vi "Mail整体图.vi"() -> ()   [LabVIEW 2014]
panel:
  in  "Check":bool
  in  "Unsubscribe":bool
  in  "Subscribe":bool
  in  "Signature":bool
  in  "Sign":bool
  in  "Send":bool
  in  "Reply":bool
  in  "Reply all":bool
  in  "Queue":bool
  in  "Post":bool
  in  "Node":bool
  in  "News":bool
  in  "New":bool
  in  "New font":bool
  in  "Mailbox":bool
  in  "Mail":bool
  in  "Log":bool
  in  "Get":bool
  in  "Generic":bool
  in  "Forward":bool
  in  "Fonts":bool
  in  "Find":bool
  in  "Email":bool
  in  "Delete":bool
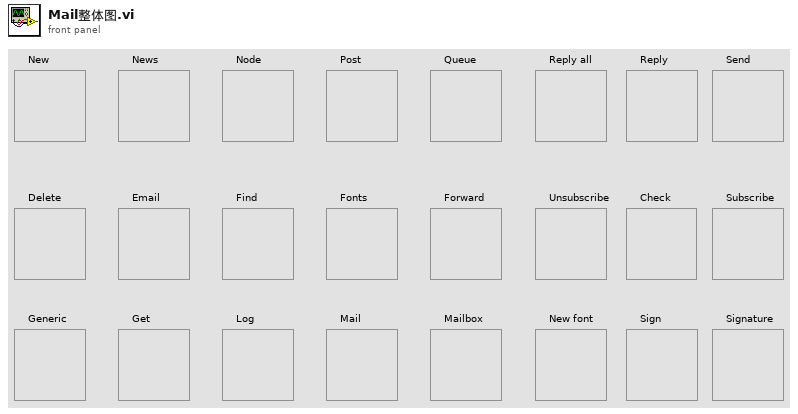
[diagram p1: front panel]
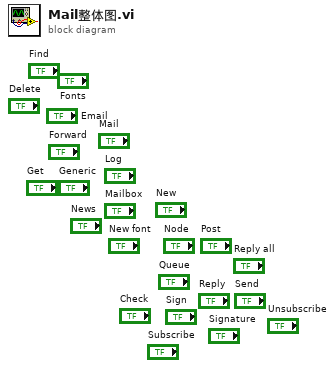
[diagram p0: block diagram]
diagram:
